vi "查找分割栏引用.vi"(8 "错误输入":errorcluster caption="错误输入（无错误）", 10 "分隔栏名字":string, 11 "引用":refnum<vi>) -> (0 "错误输出":errorcluster caption="error out", 3 "分隔栏引用":refnum<vi>)   [LabVIEW 8.6, in "窗口操作.lvlib"]
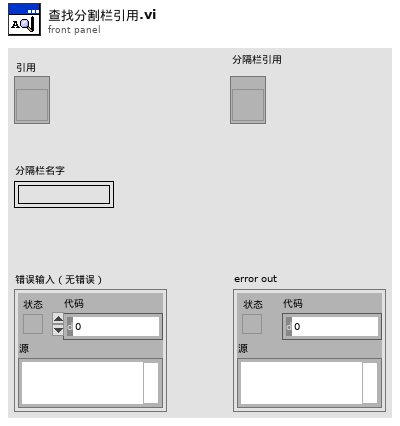
[diagram p1: front panel]
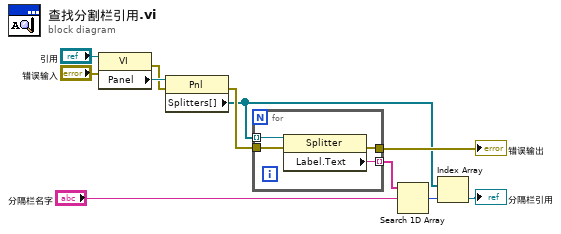
[diagram p0: block diagram]
diagram:
  n1 = property class="VI"(reference="引用", error in="错误输入") -> (error out=w9:errorcluster, "Panel"=w11:refnum<vi>)  [unwired: 1 out]
  n2 = property class="Pnl"(reference=w11, error in=w9) -> (error out=w7:errorcluster, "Splitters[]"=w2:refnum<vi>[])  [unwired: 1 out]
  n3 = for {
    tunnel: w2 -> [w15] mode=indexing
    tunnel: [w14] -> w5 mode=indexing
    tunnel: w7 -> [w13]
    tunnel: [w12] -> w6
    n4 = property class="Splitter"(reference=w15, error in=w13) -> (error out=w12:errorcluster, "Label.Text"=w14:string)  [unwired: 1 out]
  }
  "错误输出" <- w6
  n5 = Search 1D Array(1D array=w5, element="分隔栏名字") -> (index of element=w3:i32)  [unwired: 1 in]
  n6 = Index Array(array=w2, index=w3) -> (element=→"分隔栏引用":refnum<vi>)
